vi "experiment_settings.vi"() -> (0 "error out":errorcluster, 3 "Notifier out":refnum<notifier>)   [LabVIEW 2013]
uses:
  main_machine/type_defs/experiment_settings.ctl
  main_machine/type_defs/experiment_states.ctl
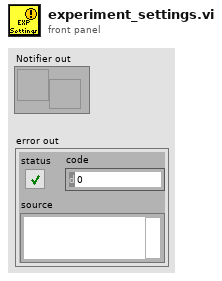
[diagram p1: front panel]
types:
  T1 = typedef "experiment_settings.ctl" = cluster{"fcs file byte offset":i64, "LED Device Handle Out":u32, "START TIME":timestamp, "CURRENT VALVE":u32, "SAMPLE #":i32, "FCS FILE PATH":path, "TIME POINT":i32, "STATE":T2, "TIME TILL SAMPLE":dbl, "DILUTION  TABLE":dbl[][]}
  T2 = typedef "experiment_states.ctl" = enum16{"OUTGROWTH", "INDUCTION", "EXPERIMENT"}
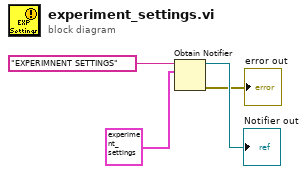
[diagram p0: block diagram]
diagram:
  n1 = Obtain Notifier(name (unnamed)="EXPERIMNENT SETTINGS", notification data type=T1 {"fcs file byte offset"=0, "LED Device Handle Out"=0, "START TIME"=timestamp(0 s since 1904-01-01), "CURRENT VALVE"=0, "SAMPLE #"=-1, "FCS FILE PATH"=path "", "TIME POINT"=0, "STATE"=enum."OUTGROWTH", "TIME TILL SAMPLE"=0.0, "DILUTION  TABLE"=[]}) -> (notifier out=→"Notifier out":refnum<notifier>, error out=→"error out":errorcluster)  [unwired: 2 in, 1 out]
